vi "DER_SetPointF_subTest.vi"(7 "Test Result in":T2=enum."Success", 8 "error in":errorcluster, 9 "DeviceID":T1, 10 "MicrogridID":u8, 11 "Message Enqueuer in":refnum<class "Message Enqueuer.lvclass">) -> (0 "error out":errorcluster, 1 "dup DeviceID":T1, 2 "dup MicrogridID":u8, 3 "Message Enqueuer out":refnum<class "Message Enqueuer.lvclass">, 5 "Test Result out":T2=enum."Success")   [LabVIEW 2018, in "IED Test Framework.lvlib" / "IED Test.lvclass"]
uses:
  IED Test.lvclass
  <vilib>/ActorFramework/Message Enqueuer/Message Enqueuer.lvclass
  Controls/Test Result.ctl
  <vilib>/ORNL/CSEISMIC DDS/CSEISMIC DDS Base/Data Types/Controls/DeviceID.ctl
  <vilib>/ORNL/CSEISMIC DDS/CSEISMIC DDS Base/Data Types/DER_SetPointF.ctl
  <vilib>/ORNL/CSEISMIC DDS/CSEISMIC DDS Base/CSEISMIC DDS.lvclass/CSEISMIC DDS.ctl
  DER Actor/DER Messages/Write DER SetpointF Msg/Write DER SetpointV Msg/Write DER SetpointF Msg.lvclass/Write DER SetpointF Msg.ctl
  <vilib>/ActorFramework/Message Enqueuer/Message Enqueuer.lvclass/Message Enqueuer.ctl
  <vilib>/ORNL/CSEISMIC DDS/CSEISMIC DDS Base/Accessors/Write DDS Reference.vi
  <vilib>/ORNL/CSEISMIC DDS/CSEISMIC DDS Base/Accessors/Read DDS Reference.vi
  <vilib>/ActorFramework/Message Enqueuer/Enqueue.vi
  <vilib>/ORNL/CSEISMIC DDS/DDS Reader/DDS Reader.lvclass
  C:/Program Files (x86)/National Instruments/LabVIEW 2018/vi.lib/ORNL/CSEISMIC DDS/CSEISMIC DDS Base/CSEISMIC DDS.lvclass
  DER Actor/DER Messages/Write DER SetpointF Msg/Write DER SetpointV Msg/Write DER SetpointF Msg.lvclass
  C:/Program Files (x86)/National Instruments/LabVIEW 2018/vi.lib/ActorFramework/Message/Message.lvclass
  <vilib>/ORNL/CSEISMIC DDS/CSEISMIC DDS Base/Error Handler.vi
  <vilib>/ActorFramework/Message Priority Queue/Priority Enqueue.vi
  <vilib>/ORNL/CSEISMIC DDS/CSEISMIC DDS Base/CSEISMIC DDS.lvclass
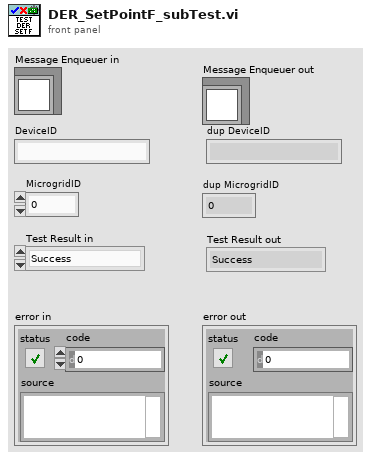
[diagram p1: front panel]
types:
  T1 = typedef "CSEISMIC DDS.lvlib/CSEISMIC DDS.lvclass/DeviceID.ctl" = string
  T2 = typedef "IED Test Framework.lvlib/IED Test.lvclass/Test Result.ctl" = enum16{"Invalid", "Success", "Failure", "Error", "Timeout"}
  T3 = typedef "CSEISMIC DDS.lvlib/CSEISMIC DDS.lvclass/DER_SetPointF.ctl" = cluster{"DeviceID":T1, "Frequency (Hz)":dbl}
  T4 = typedef "LVDDS_library.lvlib/DDS Sample Info.ctl" = cluster{"DDS_SampleStateKind":enum32{"DDS_INVALID_SAMPLE_STATE", "DDS_READ_SAMPLE_STATE", "DDS_NOT_READ_SAMPLE_STATE"}, "DDS_ViewStateKind":enum32{"DDS_INVALID_SAMPLE_STATE", "DDS_NEW_VIEW_STATE", "DDS_NOT_NEW_VIEW_STATE"}, "DDS_InstanceStateKind":enum32{"DDS_INVALID_STATE", "DDS_ALIVE_INSTANCE_STATE", "DDS_NOT_ALIVE_DISPOSED_INSTANCE_STATE", "", "DDS_NOT_ALIVE_NO_WRITERS_INSTANCE_STATE"}, "sec":i32, "nanosec":u32, "valid_data":bool}
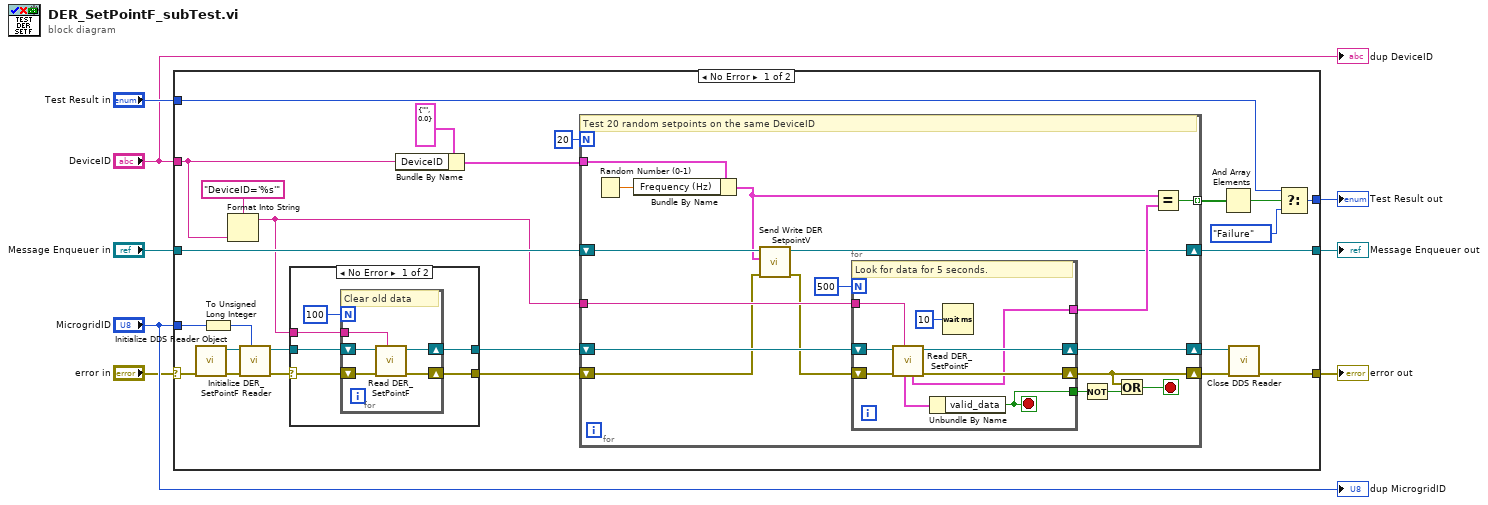
[diagram p0: block diagram]
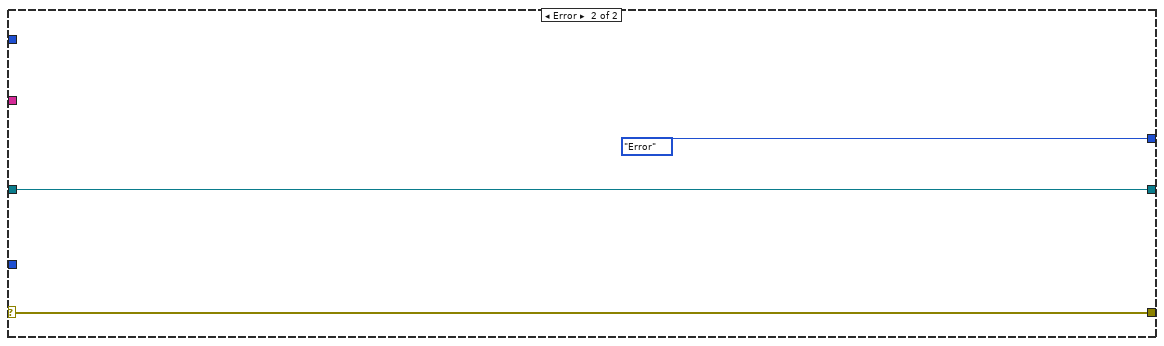
[diagram p3: hidden frame]
diagram:
  n1 = case shown="No Error" "error in" {
    selector: "error in" -> [w22 w75]
    tunnel: "Test Result in" -> [w28 _]
    tunnel: [w27 Test_Result."Error" ("f")] -> w1
    tunnel: "DeviceID" -> [w12 _]
    tunnel: "MicrogridID" -> [w18 _]
    tunnel: [w13 w75] -> w3
    tunnel: [w26 w74] -> w2
    tunnel: "Message Enqueuer in" -> [w25 w74]
    frame No Error {
      n2 = call <vilib>:"Initialize DDS Reader Object.vi"("error in"=w22) -> ("error out"=w21:errorcluster, "DDS Reader out"=w19:refnum<class "DDS Reader.lvclass">)  [unwired: 9 in]
      n3 = To Unsigned Long Integer(number=w18) -> (unsigned 32bit integer=w16:u32)
      n4 = Format Into String(format string="DeviceID='%s'", w12) -> (resulting string=w10:string)  [unwired: 2 in, 1 out]
      n5 = call <vilib>:"Initialize DER_SetPointF Reader.vi"("MicrogridID"=w16, "error in"=w21, "DDS Reader in"=w19) -> ("error out"=w20:errorcluster, "DDS Reader out"=w17:refnum<class "DDS Reader.lvclass">)  [unwired: 7 in]
      n6 = case shown="No Error" w20 {
        selector: w20 -> [w65 w72]
        tunnel: [w64 w72] -> w30
        tunnel: w17 -> [w63 w71]
        tunnel: [w62 w71] -> w24
        tunnel: w10 -> [w60 _]
        frame No Error {
          n7 = for {
            N: 100 -> [_]
            shift-right: [w70] -> w64
            shift-left: w65 -> [w67]
            shift-right: [w68] -> w62
            shift-left: w63 -> [w69]
            tunnel: w60 -> [w66]
            # "Clear old data"
            n8 = call <vilib>:"Read DER_SetPointF.vi"("Query condition"=w66, "error in"=w67, "DDS Reader in"=w69) -> ("error out"=w70:errorcluster, "DDS Reader out"=w68:refnum<class "DDS Reader.lvclass">)  [unwired: 5 in, 2 out]
          }
        }
        frame Error {
        }
      }
      n9 = Bundle By Name(cluster=T3 {"DeviceID"="", "Frequency (Hz)"=0.0} ("DER_SetPointF"), "DeviceID"=w12) -> (w11:T3)
      n10 = for {
        N: 20 -> [_]
        tunnel: w11 -> [w41]
        tunnel: [w50] -> w33 mode=indexing
        shift-right: [w47] -> w15
        shift-left: w30 -> [w36]
        shift-right: [w48] -> w14
        shift-left: w24 -> [w49]
        shift-right: [w37] -> w26
        shift-left: w25 -> [w38]
        tunnel: w10 -> [w40]
        stop <- w45 stop-if-true
        # "Test 20 random setpoints on the same DeviceID"
        n11 = Random Number (0-1)() -> (number: 0 to 1=w39:dbl)
        n12 = Bundle By Name(cluster=w41, "Frequency (Hz)"=w39) -> (w34:T3)
        n13 = call "Send Write DER SetpointV.vi"("error in"=w36, "DER_SetPointF"=w34, "Message Enqueuer"=w38) -> ("error out"=w35:errorcluster, "Message Enqueuer out"=w37:refnum<class "Message Enqueuer.lvclass">)  [unwired: 7 in]
        n14 = for {
          N: 500 -> [_]
          tunnel: [w52] -> w44
          shift-right: [w55] -> w47
          shift-left: w35 -> [w58]
          shift-right: [w56] -> w48
          shift-left: w49 -> [w57]
          tunnel: [w53] -> w46
          tunnel: w40 -> [w51]
          stop <- w53 stop-if-true
          # "Look for data for 5 seconds."
          n15 = call <vilib>:"Read DER_SetPointF.vi"("Query condition"=w51, "error in"=w58, "DDS Reader in"=w57) -> ("error out"=w55:errorcluster, "DDS Reader out"=w56:refnum<class "DDS Reader.lvclass">, "data"=w52:T3, "DDS Sample Info"=w54:T4)  [unwired: 5 in]
          n16 = Unbundle By Name(w54) -> ("valid_data"=w53:bool)
          n17 = Wait (ms)(milliseconds to wait=u32 10) -> ()  [unwired: 1 out]
        }
        n18 = Not(x=w46) -> (.not. x?=w42:bool)
        n19 = Or(x=w47, y=w42) -> (x .or. y?=w45:bool)
        n20 = Equal?(x=w34, y=w44) -> (x = y?=w50:bool)
      }
      n21 = And Array Elements(Boolean array=w33) -> (logical AND=w32:bool)
      n22 = call <vilib>:"Close DDS Reader.vi"("error in"=w15, "DDS Reader in"=w14) -> ("error out"=w13:errorcluster)  [unwired: 9 in]
      n23 = Select(t=w28, s=w32, f=Test_Result."Failure") -> (s? t:f=w27:T2)
    }
    frame Error {
    }
  }
  "Test Result out" <- w1
  "error out" <- w3
  "Message Enqueuer out" <- w2
  "dup DeviceID" <- "DeviceID"
  "dup MicrogridID" <- "MicrogridID"
